vi "BonOMM-SAOMM.Test.vi"() -> ()   [LabVIEW 2011] (continued)
                        n4610 = Subtract(x=w3202, y=w3207) -> (x-y=w3206:dbl)
                        n4611 = Absolute Value(x=w3206) -> (abs(x)=w3205:dbl)
                        n4612 = Greater?(x=w3205, y=2.0) -> (0:w3203:bool)
                        n4613 = And(x=w3208, y=w3203) -> (x .and. y?=w3209:bool)
                        n4614 = case shown="True" w3209 {
                          tunnel: w3202 -> [_ w3214]
                          frame False {
                          }
                          frame True {
                            n4615 = local read "Foyer à 0°"() -> (w3213:i32)
                            n4616 = local read "Ath_coef"() -> (w3211:dbl)
                            n4617 = To Double Precision Float(number=w3213) -> (double precision float=w3212:dbl)
                            n4618 = call "Athermalize-focus.vi"("Coefficient Thermique"=w3211, "temperature actuelle"=w3214, "Foyer à 0°"=w3212) -> ("Foyer suggérer"=w3210:i32)  [unwired: 1 in]
                            n4619 = Number To Decimal String(number=w3210) -> (decimal integer string=w3223:string)  [unwired: 1 in]
                            n4620 = Concatenate Strings("La température a suffisamment changée\npour justifier un ajustement du foyer ...\nDésirez-vous faire l'ajustement maintenant ?\n(Valeur suggérée : " ("message"), w3223, " ADU)" ("string")) -> (w3221:string)
                            n4621 = call <vilib>:"Three Button Dialog.vi"("Allow user to close window? (TRUE)"=FALSE, "Justify Message (Left)"=enum16{"Left", "Center", "Right"}."Center", "Right Button Text (\"Cancel\")"="Ne plus me demander" ("string"), "Center Button Text (\"No\")"="NON" ("string"), "Left Button Text (\"Yes\")"="OUI" ("string"), "message"=w3221) -> ("Which Button?"=w3220:T59)  [unwired: 5 in]
                            n4622 = case shown="\"Center Button\"" w3220 {
                              frame "Left Button", Default {
                              }
                              frame "Center Button" {
                                n4623 = local read "indic-T-struct"() -> (w3225:dbl)
                                n4624 = local write "tmp.str"(w3225) -> ()
                              }
                              frame "Right Button" {
                                "Bypass Auto-focus" <- TRUE ("Allow user to close window? (TRUE)")
                              }
                            }
                          }
                        }
                      }
                    }
                  }
                }
                n4625 = Quotient & Remainder(x=w3171, y=10) -> (x-y*floor(x/y)=w3173:i32)  [unwired: 1 out]
                n4626 = Equal To 0?(x=w3173) -> (x = 0?=w3170:bool)
                n4627 = case shown="False" w3170 {
                  frame False {
                  }
                  frame True {
                    n4628 = disable-structure shown="Enabled" {
                      frame Disabled {
                        n4629 = call "DCON-Read.vi"("VRN in"="HexTemp VRN") -> ("DataCluster"=→"Hexapode Temperatures":T13, "Boolean array"=→"Hexapod Alarms":bool[], "error out"=w3177:errorcluster)  [unwired: 11 in, 1 out]
                        n4630 = local write "HexapodeTempError"(w3177) -> ()
                        n4631 = Unbundle By Name(w3177) -> ("status"=w3180:bool)
                        n4632 = Not(x=w3180) -> (.not. x?=→"HexTemp COMM":bool)
                      }
                      frame Enabled {
                      }
                    }
                  }
                }
              }
              event "Setting", "Focus slew": Value Change {
                n4633 = event-data() -> ()  [unwired: 1 in, 6 out]
                n4634 = local read "Focus slew"() -> (w3229:bool)
                n4635 = local read "Setting"() -> (w3231:bool)
                n4636 = Not(x=w3229) -> (.not. x?=w3228:bool)
                n4637 = case shown="False" w3231 {
                  selector: w3231 -> [_ w3237]
                  tunnel: [w3232 w3237] -> w3230
                  frame False {
                    n4638 = local read "Foyer"() -> (w3235:dbl)
                    n4639 = local read "Foyer Nominal"() -> (w3236:dbl)
                    n4640 = Subtract(x=w3236, y=w3235) -> (x-y=w3234:dbl)
                    n4641 = Greater?(x=w3234, y=1.0) -> (0:w3232:bool)
                  }
                  frame True {
                  }
                }
                n4642 = And(x=w3228, y=w3230) -> (x .and. y?=w3227:bool)
                n4643 = case shown="False" w3227 {
                  frame False {
                    # "Ici, normalement, on est à la fin d'une séquence de foyer ..."
                    n4644 = local read "Foyer"() -> (w3238:dbl)
                    n4645 = Get Date/Time In Seconds() -> (seconds since 1Jan1904=w3240:timestamp)
                    n4646 = To Extended Precision Float(1:w3240) -> (0:→"last_foc_chg":ext)
                    n4647 = local write "Foyer Nominal"(w3238) -> ()
                    n4648 = local read "indic-T-struct"() -> (→"tmp.str":dbl)
                    "CheckFocus" <- TRUE
                  }
                  frame True {
                  }
                }
              }
              event "Recalculer": Value Change {
                # "Ne devrait pas être fait sur une base régulière, mais simplement quand les paramètres ont changés ...\n\nC'est ici qu'on veut cleaner les dossiers de data et construire les mosaiques d'image et de données !!!\n\nPour l'instant, tout a été arraché le temps de débuggé les Queries USNO & DSS !!!"
                n4649 = event-data() -> ()  [unwired: 1 in, 6 out]
                n4650 = case shown="True" "Recalculer" {
                  selector: "Recalculer" -> [_ w3250]
                  frame False {
                  }
                  frame True {
                    n4651 = stacked-sequence {
                      seq-local: [w3257 _ _ _] -> [_ w3261 w3289 _]
                      seq-local: [w3256 _ _ _] -> [_ w3262 w3288 _]
                      tunnel: w3250 -> [_ _ _ _]
                      frame #0 {
                        w3258 = FALSE ("DSS_ready")
                        # "Époque DSS et USNO"
                        # "Ici il faudra s'assurer que l'astrométrie tourne autour du centre, mais\nutilise la position synchronisée comme valeur de référence"
                        # "Ces variables sont probablement\nmaintenant inutiles"
                        # "à remettre éventuellement ..."
                        # "Calcul les paramètres du champ ..."
                        n4652 = disable-structure shown="Disabled" {
                          frame Disabled {
                          }
                          frame Enabled {
                          }
                        }
                        n4653 = local read "Img DEC"() -> (w3253:dbl)
                        n4654 = local read "Img RA"() -> (w3252:dbl)
                        n4655 = local read "Epoch Tel"() -> (w3255:dbl)
                        n4656 = call "precess.vi"("Eq2"=2000.0, "Eq1"=w3255, "DEC 1"=w3253, "RA 1"=w3252) -> ("DEC 2"=w3257:dbl, "RA 2"=w3256:dbl)
                        n4657 = local write "USNO_ready"(FALSE) -> ()
                        n4658 = local write "Indicateur d'état"("Calcul des paramètres du champ") -> ()
                        "DSS_ready" <- w3258
                        "USNO_ready" <- w3258
                      }
                      frame #1 {
                        # "Télécharge les données USNO associées ..."
                        # "DEC centre img"
                        # "RA centre img"
                        n4659 = flat-sequence {
                          tunnel: w3262 -> [w3272]
                          tunnel: w3261 -> [w3271]
                          tunnel: [w3266] -> w3260
                          tunnel: w3260 -> [w3284]
                          frame #0 {
                            # "R1mag limite USNO"
                            n4660 = local read "Représentation"() -> (w3263:dbl)
                            n4661 = local read "path_data"() -> (w3268:path)
                            n4662 = while {
                              stop <- w3274 stop-if-true
                              n4663 = local read "BestTargetLed"() -> (w3276:bool)
                              n4664 = Wait (ms)(milliseconds to wait=u32 333) -> ()  [unwired: 1 out]
                              n4665 = Not(x=w3276) -> (.not. x?=w3275:bool)
                              n4666 = local write "BestTargetLed"(w3275) -> ()
                              n4667 = local read "USNO_ready"() -> (w3274:bool)
                            }
                            n4668 = local read "wgetexec"() -> (w3267:path)
                            n4669 = call "QueryUSNO.vi"("wget"=w3267, "Data dir Path"=w3268, "mag_limit"=12.0, "radius"=w3263, "DEC"=w3271, "RA"=w3272) -> ("Data OUT"=w3269:string[][], "No Error"=w3264:bool)  [unwired: 3 in, 1 out]
                            n4670 = case shown="True" w3264 {
                              tunnel: w3269 -> [_ w3283]
                              tunnel: w3264 -> [w3278 w3280]
                              tunnel: [w3278 w3280] -> w3266
                              tunnel: [TRUE TRUE] -> w3265
                              frame False {
                              }
                              frame True {
                                # "6 = R1mag"
                                n4671 = call "Sort_USNO_data.vi"("Column Used"=6, "Data IN"=w3283) -> ("Data OUT"=→"USNO_data":string[][])  [unwired: 8 in, 1 out]
                              }
                            }
                            n4672 = local write "USNO_ready"(w3265) -> ()
                          }
                          frame #1 {
                            n4673 = local write "USNO_ready"(w3284) -> ()
                            n4674 = local write "BestTargetLed"(w3284) -> ()
                          }
                        }
                      }
                      frame #2 {
                        # "Pour que l'image disparaisse quand\non coche ou décoche l'option du menu"
                        # "Get the dss image ...\nÉventuellement va vérifier l'existence et créer les mosaïques\nPour l'instant, on ne le permet qu'avec le bouton \"GetDSS\""
                        n4675 = local read "Img RA"() -> (w3299:dbl)
                        n4676 = local read "imageDSS"() -> (w3286:bool)
                        n4677 = local read "Img DEC"() -> (w3290:dbl)
                        n4678 = Subtract(x=w3288, y=w3299) -> (x-y=w3297:dbl)
                        n4679 = Subtract(x=w3289, y=w3290) -> (x-y=w3298:dbl)
                        n4680 = Absolute Value(x=w3297) -> (abs(x)=w3296:dbl)
                        n4681 = Absolute Value(x=w3298) -> (abs(x)=w3295:dbl)
                        n4682 = Greater?(x=w3296, y=1.0) -> (0:w3291:bool)
                        n4683 = Not(x=w3286) -> (.not. x?=w3285:bool)
                        n4684 = Greater?(x=w3295, y=1.0) -> (0:w3292:bool)
                        n4685 = Compound Arithmetic op=OR(w3291, w3292, w3285) -> (w3287:bool)
                        n4686 = case shown="True" w3287 {
                          tunnel: w3288 -> [_ w3302]
                          tunnel: w3289 -> [_ w3303]
                          frame False {
                            n4687 = local read "imageDSS"() -> (w3300:bool)
                            n4688 = local write "DSS_ready"(w3300) -> ()
                          }
                          frame True {
                            n4689 = local read "imageDSS"() -> (w3301:bool)
                            n4690 = case shown="True" w3301 {
                              tunnel: w3303 -> [_ w3308]
                              tunnel: w3302 -> [_ w3307]
                              frame False {
                                n4691 = property on="TableXYPos" class="XYGraph (strict)"("PlotImages.Back"=picture data[5B] ("Images")) -> ()  [unwired: 2 in, 2 out]
                              }
                              frame True {
                                n4692 = flat-sequence {
                                tunnel: w3307 -> [w3318]
                                tunnel: w3308 -> [w3319]
                                tunnel: [w3319] -> w3306
                                tunnel: [w3318] -> w3305
                                tunnel: w3306 -> [w3328]
                                tunnel: w3305 -> [w3327]
                                frame #0 {
                                w3309 = u16 1 items=["Region d'intérêt", "Prévisualisation"] ("ImageUsage")
                                w3314 = 0
                                n4693 = Initialize Array(sgl 0.0, w3314, w3314) -> (w3313:sgl[][])
                                n4694 = local write "ImgData"(w3313) -> ()
                                n4695 = local write "SubIMG4DSS?"(TRUE ("SubIMG4DSS?")) -> ()
                                n4696 = local write "ImgAstrom"(T4 {"NAXIS"=[], "CD"=[], "CDELT"=[], "CRPIX"=[], "CTYPE"=[], "CRVAL"=[], "LONGPOLE"=180.0, "LATPOLE"=90.0, "PV2"=[]} ("ImgAstrom")) -> ()
                                n4697 = call "Draw_crosshair.vi"("Image IN"=w3313, "White Value"=sgl 255.0) -> ("Image OUT"=w3312:sgl[][])  [unwired: 13 in]
                                n4698 = property on="TableXYPos" class="XYGraph (strict)"("PlotImages.Back"=picture data[5B] ("Images")) -> ()  [unwired: 2 in, 2 out]
                                n4699 = local write "subimg"(w3312) -> ()
                                n4700 = local write "ImageUsage"(w3309) -> ()
                                }
                                frame #1 {
                                # "Ici, le code devrait vérifier l'existence des images sur le disque ..."
                                n4701 = local read "Représentation"() -> (w3322:dbl)
                                n4702 = local read "path_dss"() -> (w3325:path)
                                n4703 = local read "wgetexec"() -> (w3324:path)
                                n4704 = Add(x=4.0, y=w3322) -> (x+y=w3320:dbl)
                                n4705 = call "Query_Vizier.vi"("Folder"=w3325, "wget"=w3324, "Width"=w3320, "Height"=w3320, "DEC"=w3328, "RA"=w3327) -> ("error?"=w3323:bool, "Path2Image"=w3331:path)  [unwired: 4 in]
                                "Path2Image" <- w3331
                                n4706 = case shown="False" w3323 {
                                tunnel: w3327 -> [w3336 _]
                                tunnel: w3328 -> [w3335 _]
                                tunnel: w3331 -> [w3338 _]
                                tunnel: [w3336 -inf ("RA OUT")] -> w3330
                                tunnel: [w3335 -inf ("RA OUT")] -> w3329
                                tunnel: [TRUE FALSE] -> w3326
                                frame False {
                                # "ImgData et ImgAstrom\nsont lié à plus grand que le\nchamp affiché."
                                n4707 = local read "FieldAstrom"() -> (w3334:T4)
                                n4708 = property on="TableXYPos" class="XYGraph (strict)"() -> ("Height"=w3344:u32, "Width"=w3343:u32)  [unwired: 2 in, 2 out]
                                n4709 = property on="TableXYPos" class="XYGraph (strict)"() -> ("XScale.Range"=w3340:T26, "YScale.Range"=w3339:T26)  [unwired: 2 in, 2 out]
                                n4710 = To Long Integer(number=w3344) -> (32bit integer=w3342:i32)
                                n4711 = To Long Integer(number=w3343) -> (32bit integer=w3341:i32)
                                n4712 = call "Draw_graph_background.vi"("Y Scale.Range"=w3339, "ImgRA"=w3336, "X Scale.Range"=w3340, "ImgDEC"=w3335, "Field Astrometry"=w3334, "New Width"=w3341, "New Height"=w3342, "path"=w3338) -> ("ImgData"=→"ImgData":sgl[][], "Astrometry"=→"ImgAstrom":T4, "Images"=w3333:picture)  [unwired: 1 out]
                                n4713 = property on="TableXYPos" class="XYGraph (strict)"("PlotImages.Back"=w3333) -> ()  [unwired: 2 in, 2 out]
                                }
                                frame True {
                                }
                                }
                                "Img RA" <- w3330
                                "Img DEC" <- w3329
                                n4714 = local write "DSS_ready"(w3326) -> ()
                                }
                                }
                              }
                            }
                          }
                        }
                      }
                      frame #3 {
                        # "Retrace l'image de la caméra de référence ..."
                        n4715 = local write "Recalculer"(FALSE ("Recalculer")) -> ()
                      }
                    }
                  }
                }
                n4716 = while {
                  tunnel: [FALSE] -> w3243
                  stop <- w3249 continue-if-true
                  n4717 = local read "Downloading ..."() -> (w3247:bool)
                  n4718 = Not(x=w3247) -> (.not. x?=→"Downloading ...":bool)
                  n4719 = Wait (ms)(milliseconds to wait=u32 333) -> ()  [unwired: 1 out]
                  n4720 = local read "Recalculer"() -> (w3249:bool)
                }
                n4721 = local write "Downloading ..."(w3243) -> ()
              }
              event "Slewing": Value Change {
                n4722 = event-data() -> ("NewVal"=w3350:bool)  [unwired: 1 in, 5 out]
                n4723 = case shown="False" w3350 {
                  frame False {
                    w3352 = FALSE ("Blinking")
                    w3353 = 0
                    # "Fin d'un déplacement ..."
                    # "Activer les boutons"
                    n4724 = property on="GO" class="Bool (strict)"("Disabled"=w3353) -> ()  [unwired: 2 in, 2 out]
                    n4725 = property on="Synctel" class="Bool (strict)"("Disabled"=w3353) -> ()  [unwired: 2 in, 2 out]
                    n4726 = property on="ModifRotation" class="Bool (strict)"("Disabled"=w3353) -> ()  [unwired: 2 in, 2 out]
                    n4727 = property on="Offset OK" class="Bool (strict)"("Disabled"=w3353) -> ()  [unwired: 2 in, 2 out]
                    n4728 = property on="ModifFoyer" class="Bool (strict)"("Disabled"=w3353) -> ()  [unwired: 2 in, 2 out]
                    n4729 = property on="Écran" class="Bool (strict)"("Disabled"=w3353) -> ()  [unwired: 2 in, 2 out]
                    n4730 = property on="Zénith" class="Bool (strict)"("Disabled"=w3353) -> ()  [unwired: 2 in, 2 out]
                    n4731 = property on="Range" class="Bool (strict)"("Disabled"=w3353) -> ()  [unwired: 2 in, 2 out]
                    n4732 = property on="Zénith" class="Bool (strict)"("Blinking"=w3352) -> ()  [unwired: 2 in, 2 out]
                    n4733 = property on="Range" class="Bool (strict)"("Blinking"=w3352) -> ()  [unwired: 2 in, 2 out]
                    n4734 = property on="Écran" class="Bool (strict)"("Blinking"=w3352) -> ()  [unwired: 2 in, 2 out]
                    n4735 = property on="ModCoor" class="Bool (strict)"("Disabled"=w3353) -> ()  [unwired: 2 in, 2 out]
                    n4736 = property on="ModifDome" class="Bool (strict)"("Disabled"=w3353) -> ()  [unwired: 2 in, 2 out]
                    n4737 = local read "Déplacement usager"() -> (w3351:bool)
                    n4738 = case shown="True" w3351 {
                      frame False {
                        w3354 = FALSE ("Déplacement usager")
                        n4739 = local write "Déplacement usager"(w3354) -> ()
                        n4740 = local write "From library"(w3354) -> ()
                      }
                      frame True {
                        w3363 = "\t"
                        w3369 = "_"
                        w3375 = TRUE ("replace all? (F)")
                        w3376 = " "
                        w3377 = "0"
                        w3380 = i16 2 ("width (-)")
                        w3381 = i16 0 ("width (-)")
                        # "Devrait aussi être mis dans un log pour pouvoir y revenir plus tard ..."
                        # "Enregistre la nouvelle position du télescope"
                        n4741 = local write "Déplacement usager"(FALSE ("Déplacement usager")) -> ()
                        n4742 = local read "Epoch Tel"() -> (w3385:dbl)
                        n4743 = local read "DEC Tel"() -> (w3383:dbl)
                        n4744 = local read "RA Tel"() -> (w3384:dbl)
                        n4745 = call "time-sec-to-time-str-DEC.vi"("Numeric"=w3384) -> ("formatted-str"=w3366:string)
                        n4746 = call "time-sec-to-time-str-DEC.vi"("Numeric"=w3383) -> ("formatted-str"=w3365:string)
                        n4747 = Number To Fractional String(number=w3385, width (-)=i16 4, precision (6)=i16 2) -> (F-format string=w3364:string)  [unwired: 1 in]
                        n4748 = Get Date/Time String() -> (time string=w3367:string)  [unwired: 3 in, 1 out]
                        n4749 = local read "From library"() -> (w3389:bool)
                        n4750 = Concatenate Strings(w3367, w3363, w3366, w3363, w3365, w3363, w3364, "\r\n") -> (w3355:string)
                        n4751 = call "GetUTC.vi"() -> ("Day"=w3359:dbl, "Month"=w3360:dbl, "Year"=w3361:dbl)  [unwired: 6 out]
                        n4752 = case shown="True" w3389 {
                          tunnel: [FALSE FALSE] -> w3388
                          tunnel: w3366 -> [w3394 w3401]
                          tunnel: w3365 -> [w3393 w3402]
                          tunnel: w3364 -> [w3392 w3403]
                          tunnel: w3367 -> [w3391 w3400]
                          frame False {
                            w3396 = i16 0 items=["tel coords", "tel offset", "guidage"] ("options")
                            n4753 = local read "Obslib"() -> (w3397:string[][])
                            n4754 = Build Array(w3394, w3393, w3392, w3391) -> (w3398:string[])
                            n4755 = call "Coords to chart(new).vi"("DataLine"=w3398, "options"=w3396, "Tableau entrant"=w3397) -> ("historique"=w3399:string[][])
                            n4756 = local write "Obslib"(w3399) -> ()
                          }
                          frame True {
                            w3405 = i16 0 items=["tel coords", "tel offset", "guidage"] ("options")
                            n4757 = local read "Obslib"() -> (w3406:string[][])
                            n4758 = Build Array(w3401, w3402, w3403, w3400) -> (w3407:string[])
                            n4759 = call "Coords to chart(new).vi"("DataLine"=w3407, "options"=w3405, "Tableau entrant"=w3406) -> ("historique"=w3408:string[][])
                            n4760 = local write "Obslib"(w3408) -> ()
                          }
                        }
                        "From library" <- w3388
                        n4761 = Number To Fractional String(number=w3361, width (-)=i16 4, precision (6)=w3381) -> (F-format string=w3374:string)  [unwired: 1 in]
                        n4762 = Number To Fractional String(number=w3360, width (-)=w3380, precision (6)=w3381) -> (F-format string=w3379:string)  [unwired: 1 in]
                        n4763 = Number To Fractional String(number=w3359, width (-)=w3380, precision (6)=w3381) -> (F-format string=w3378:string)  [unwired: 1 in]
                        n4764 = Search and Replace String(replace all?=w3375, input string=w3379, search string=w3376, replace string=w3377) -> (result string=w3373:string)  [unwired: 4 in, 3 out]
                        n4765 = Search and Replace String(replace all?=w3375, input string=w3378, search string=w3376, replace string=w3377) -> (result string=w3372:string)  [unwired: 4 in, 3 out]
                        n4766 = local read "path_pointing"() -> (w3371:path)
                        n4767 = Concatenate Strings(w3374, w3369, w3373, w3369, w3372, ".pnt") -> (w3370:string)
                        n4768 = Build Path(base path=w3371, name or relative path=w3370) -> (appended path=w3356:path)
                        n4769 = local read "File I/O Error"() -> (w3358:errorcluster)
                        n4770 = call "PNT-Data-Write.vi"("Path IN"=w3356, "Data Line"=w3355, "Error IN"=w3358) -> ("Error OUT"=w3357:errorcluster)  [unwired: 11 in, 1 out]
                        n4771 = local write "File I/O Error"(w3357) -> ()
                      }
                    }
                  }
                  frame True {
                    w3409 = 2
                    # "Début d'un déplacement"
                    # "Désactiver les boutons de TCS"
                    n4772 = property on="GO" class="Bool (strict)"("Disabled"=w3409) -> ()  [unwired: 2 in, 2 out]
                    n4773 = property on="ModifFoyer" class="Bool (strict)"("Disabled"=w3409) -> ()  [unwired: 2 in, 2 out]
                    n4774 = property on="Écran" class="Bool (strict)"("Disabled"=w3409) -> ()  [unwired: 2 in, 2 out]
                    n4775 = property on="ModCoor" class="Bool (strict)"("Disabled"=w3409) -> ()  [unwired: 2 in, 2 out]
                    n4776 = property on="Zénith" class="Bool (strict)"("Disabled"=w3409) -> ()  [unwired: 2 in, 2 out]
                    n4777 = property on="Range" class="Bool (strict)"("Disabled"=w3409) -> ()  [unwired: 2 in, 2 out]
                    n4778 = property on="Synctel" class="Bool (strict)"("Disabled"=w3409) -> ()  [unwired: 2 in, 2 out]
                    n4779 = property on="ModifRotation" class="Bool (strict)"("Disabled"=w3409) -> ()  [unwired: 2 in, 2 out]
                    n4780 = property on="Offset OK" class="Bool (strict)"("Disabled"=w3409) -> ()  [unwired: 2 in, 2 out]
                    n4781 = property on="ModifDome" class="Bool (strict)"("Disabled"=w3409) -> ()  [unwired: 2 in, 2 out]
                  }
                }
              }
            }
            n4782 = local read "Quit"() -> (w3167:bool)
          }
          "Événements Software" <- w952
          n4783 = while {
            tunnel: [w1226] -> w950
            stop <- w1226 stop-if-true
            # "Boucle périodique pour PrAMS + Hexapode + LVDTs\nÉvénements lents ..."
            n4784 = stacked-sequence {
              frame #0 {
                n4785 = disable-structure shown="Disabled" {
                  frame Disabled {
                    n4786 = local read "LVDT-RA"() -> (w1230:refnum<k21>)
                    n4787 = local read "LVDT Error"() -> (w1229:errorcluster)
                    n4788 = Unbundle By Name(w1229) -> ("status"=w1228:bool)
                    n4789 = case shown="False" w1228 {
                      tunnel: w1230 -> [w1243 _]
                      tunnel: w1229 -> [_ _]
                      frame False {
                        n4790 = call "Read-LVDT-Data.vi"("shared variable refnum"=w1243, "MaxLen"=631 ("timeout ms"), "Data IN"="LVDT-RA-Data") -> ("Graph Data"=w1237:dbl[], "Data OUT"=w1239:dbl[], "error out"=→"LVDT Error":errorcluster)  [unwired: 10 in]
                        "Graph Data" <- w1237
                        n4791 = local write "LVDT-RA-Data"(w1239) -> ()
                        n4792 = Subtract(x=w1237, y="LVDT-zero") -> (x-y=w1244:dbl[])
                        n4793 = Multiply(x="LVDT-scale", y=w1244) -> (x*y=w1234:dbl[])
                        n4794 = Array Size(array=w1234) -> (size(s)=w1233:i32)
                        n4795 = Decrement(x=w1233) -> (x-1=w1231:i32)
                        n4796 = Bundle(0.0, "LVDT-time"="LVDT-time", w1234) -> (→"LVDT-RA-coarse" →"LVDT-RA-closeup":cluster{dbl, "LVDT-time":dbl, dbl[]})  [unwired: 1 in]
                        n4797 = Index Array(array=w1234, index=w1231) -> (element=→"LVDT-RA-inst":dbl)
                      }
                      frame True {
                      }
                    }
                  }
                  frame Enabled {
                  }
                }
              }
              frame #1 {
                # "Si la communication avec TCS et PrAMS sont actives, on update les valeurs de ALT/AZ/ROT de Prams\n\nN.B. : L'erreur associée (#64) : est ignorée par la boucle \"emterror\" ci-bas ..."
                n4798 = local read "PrAMS COMM"() -> (w1248:bool)
                n4799 = local read "TCS COMM"() -> (w1249:bool)
                n4800 = And(x=w1249, y=w1248) -> (x .and. y?=w1247:bool)
                n4801 = case shown="False" w1247 {
                  frame False {
                  }
                  frame True {
                    n4802 = local read "Epoch Tel"() -> (w1263:dbl)
                    n4803 = local read "RA Tel"() -> (w1267:dbl)
                    n4804 = local read "DEC Tel"() -> (w1266:dbl)
                    n4805 = local read "AnnéeRL"() -> (w1262:dbl)
                    n4806 = local read "LST"() -> (w1261:dbl)
                    n4807 = call "ad2deg.vi"("DEC (sec)"=w1266, "RA (sec)"=w1267) -> ("DEC (°)"=w1264:dbl, "RA (°)"=w1265:dbl)
                    n4808 = call "ad2deg.vi"("RA (sec)"=w1261) -> ("RA (°)"=w1260:dbl)  [unwired: 1 in, 1 out]
                    n4809 = call "precess.vi"("Eq2"=w1262, "Eq1"=w1263, "DEC 1"=w1264, "RA 1"=w1265) -> ("DEC 2"=w1258:dbl, "RA 2"=w1268:dbl)
                    "DEC" <- w1258
                    n4810 = Subtract(x=w1260, y=w1268) -> (x-y=w1259:dbl)
                    "HA" <- w1259
                    n4811 = control-ref of="PrAMS-ACK"() -> (w1253:refnum<vi>)
                    n4812 = control-ref of="PrAMS actif"() -> (w1252:refnum<vi>)
                    n4813 = local read "PrAMS VRN"() -> (w1254:refnum<visa-resource-name>)
                    n4814 = local read "PrAMS Error"() -> (w1255:errorcluster)
                    n4815 = local read "Signature"() -> (w1257:u32)
                    n4816 = local read "MessageType"() -> (w1256:cluster{string[], u32[]})
                    n4817 = call "SAOMM-SetTelescopeProperties.vi"("PRAMMS-COMM IN"=w1254, "PramsActif"=w1252, "PrAMS-ACK"=w1253, "HA"=w1259, "DEC"=w1258, "Error IN"=w1255, "Signature"=w1257, "MsgTypeEnum"=w1256) -> ("PRAMMS-COMM OUT"=w1250:refnum<visa-resource-name>, "Error OUT"=w1251:errorcluster)  [unwired: 6 in]
                    n4818 = local write "PrAMS VRN"(w1250) -> ()
                    n4819 = local write "PrAMS Error"(w1251) -> ()
                  }
                }
              }
              frame #2 {
                # "L'angle ne peut être envoyé que si l'asservissement est OFF"
                n4820 = local read "Servo"() -> (w1269:bool)
                n4821 = case shown="False" w1269 {
                  frame False {
                    # "Prams à un 180° dans sa matrice d'Euler"
                    n4822 = local read "RotationEffective"() -> (w1280:dbl)
                    n4823 = local read "PrAMS VRN"() -> (w1275:refnum<visa-resource-name>)
                    n4824 = control-ref of="PrAMS-ACK"() -> (w1272:refnum<vi>)
                    n4825 = local read "PrAMS Error"() -> (w1276:errorcluster)
                    n4826 = local read "MessageType"() -> (w1277:cluster{string[], u32[]})
                    n4827 = control-ref of="PrAMS actif"() -> (w1273:refnum<vi>)
                    n4828 = local read "Signature"() -> (w1274:u32)
                    n4829 = call "Fix_angle.vi"("±180 -> 0-360?"=FALSE, "Angle IN"=w1280) -> ("Angle OUT"=w1279:dbl)  [unwired: 3 in]
                    n4830 = Negate(x=w1279) -> (-x=w1270:dbl)
                    n4831 = call-poly "SAOMM-Num2littleEndian.vi"("Number"=w1270) -> ("LiitleEndianedData"=w1278:u8[])  [unwired: 14 in]
                    n4832 = call "SAOMM-SendSET.vi"("PRAMMS-COMM IN"=w1275, "Active Refnum"=w1273, "PrAMS-ACK"=w1272, "Signature"=w1274, "Error IN"=w1276, "MessageType"=w1277, "Active SET"="emtSetMountingPlateAngle", "Value (little endianed byte array)"=w1278) -> ()  [unwired: 4 in, 4 out]
                  }
                  frame True {
                  }
                }
              }
              frame #3 {
                # "Enregistre environ 2 fois par \"Considered Lenght\""
                # "Update l'historique de guidage et enregistre log dans un fichier ..."
                n4833 = local read "Graph-Centroids"() -> (w1284:cluster{"TimeArray":dbl[], dbl[]}[])
                n4834 = Index Array(array=w1284) -> (element #1=w1301:cluster{"TimeArray":dbl[], dbl[]}, element #2=w1300:cluster{"TimeArray":dbl[], dbl[]})  [unwired: 2 in]
                n4835 = Unbundle(w1301) -> (w1298:dbl[])  [unwired: 1 out]
                n4836 = Unbundle(w1300) -> ("TimeArray"=w1283:dbl[], w1299:dbl[])
                n4837 = local read "LastSaveTimeStamp"() -> (w1290:dbl)
                n4838 = local read "ConsideredLenght"() -> (w1294:i32)
                n4839 = call "TimeStamp-Extractor.vi"("TimeStampArray"=w1283) -> ("LastTimestamp"=w1289:dbl)  [unwired: 12 in, 2 out]
                n4840 = To Double Precision Float(number=w1294) -> (double precision float=w1293:dbl)
                n4841 = call "Guide_error_histo.vi"("X Array"=w1298, "intervals"=11, "Y array"=w1299, "limite haute"=5.0, "limite basse"=-5.0 ("limite haute")) -> ("XY graph"=→"Guiderreur":cluster{dbl[], dbl[]}[])  [unwired: 1 out]
                n4842 = local read "CentroidsData"() -> (w1285:cluster{dbl[], dbl[]}[])
                n4843 = expression code="x/2"(w1293) -> (w1292:dbl)
                n4844 = Add(x=w1290, y=w1292) -> (x+y=w1291:dbl)
                n4845 = Greater?(x=w1289, y=w1291) -> (0:w1287:bool)
                n4846 = Or(x="ForceSaveToFile", y=w1287) -> (x .or. y?=w1288:bool)
                n4847 = case shown="True" w1288 {
                  tunnel: w1289 -> [_ w1328]
                  tunnel: w1290 -> [_ w1313]
                  tunnel: w1285 -> [_ w1329]
                  frame False {
                  }
                  frame True {
                    # "Va peut-être perdre les quelques minutes juste avant la fermeture \n... pour ce que ça changera c'est beaucoup de travail."
                    n4848 = local read "path_trackfile"() -> (w1312:path)
                    n4849 = Strip Path(path=w1312) -> (stripped path=w1306:path)  [unwired: 1 out]
                    n4850 = local read "path_trackfile"() -> (w1326:path)
                    n4851 = Build Path(base path=w1306, name or relative path="Hexapod") -> (appended path=w1304:path)
                    n4852 = call "GetPathFromTimeStamp.vi"("UTC Time"=FALSE, "LocalTimeStamp"=w1313, "Changement de date à midi ?"=TRUE) -> ("Date String"=w1302:string)  [unwired: 11 in, 1 out]
                    n4853 = call "CheckAndCreateDirectory.vi"("Path IN"=w1304) -> ("Path OUT"=w1303:path, "Exists?"=w1309:bool, "Created?"=w1308:bool)  [unwired: 12 in]
                    n4854 = call "GetPathFromTimeStamp.vi"("UTC Time"=TRUE, "LocalTimeStamp"=w1328, "Changement de date à midi ?"=TRUE) -> ("Date String"=w1327:string)  [unwired: 11 in, 1 out]
                    n4855 = local read "ForceSaveToFile"() -> (w1318:bool)
                    n4856 = Build Path(base path=w1326, name or relative path=w1327) -> (appended path=w1325:path)
                    n4857 = Or(x=w1309, y=w1308) -> (x .or. y?=w1307:bool)
                    n4858 = local read "Servo"() -> (w1317:bool)
                    n4859 = case shown="True" w1307 {
                      tunnel: w1313 -> [_ w1336]
                      tunnel: w1303 -> [_ w1335]
                      tunnel: w1302 -> [_ w1333]
                      frame False {
                      }
                      frame True {
                        # "Log de l'hexapode"
                        n4860 = Concatenate Strings(w1333, ".hex") -> (w1331:string)
                        n4861 = local read "HexXData"() -> (w1338:cluster{dbl[], dbl[]}[])
                        n4862 = local read "HexYData"() -> (w1337:cluster{dbl[], dbl[]}[])
                        n4863 = local read "CumulativeError"() -> (w1330:cluster{dbl[], dbl[]}[])
                        n4864 = Build Path(base path=w1335, name or relative path=w1331) -> (appended path=w1334:path)
                        n4865 = call "LogHexapodData.vi"("LogFilePath"=w1334, "TimeStampTreshold"=w1336, "X IN"=w1338, "Y IN"=w1337, "Cumul IN"=w1330) -> ()  [unwired: 10 in, 1 out]
                      }
                    }
                    n4866 = call "CheckAndCreateDirectory.vi"("Path IN"=w1325) -> ("Path OUT"=w1322:path, "Exists?"=w1324:bool, "Created?"=w1323:bool)  [unwired: 12 in]
                    n4867 = Or(x=w1324, y=w1323) -> (x .or. y?=w1320:bool)
                    n4868 = Or(x=w1317, y=w1318) -> (x .or. y?=w1316:bool)
                    n4869 = local read "TrackLogFilename"() -> (w1321:string)
                    n4870 = And(x=w1320, y=w1316) -> (x .and. y?=w1319:bool)
                    n4871 = case shown="True" w1319 {
                      tunnel: w1329 -> [_ w1348]
                      tunnel: w1313 -> [_ w1345]
                      tunnel: w1322 -> [_ w1344]
                      tunnel: w1321 -> [_ w1342]
                      frame False {
                      }
                      frame True {
                        # "Log de guidage"
                        n4872 = local read "SNRData"() -> (w1340:cluster{dbl[], dbl[]}[])
                        n4873 = local read "FluxData"() -> (w1339:cluster{dbl[], dbl[]}[])
                        n4874 = Build Path(base path=w1344, name or relative path=w1342) -> (appended path=w1343:path)
                        n4875 = local write "ForceSaveToFile"(FALSE ("ForceSaveToFile")) -> ()
                        n4876 = local read "Dec Sonde"() -> (w1347:dbl)
                        n4877 = local read "RA Sonde"() -> (w1346:dbl)
                        n4878 = call "LogSourceData.vi"("LogFilePath"=w1343, "DECsonde"=w1347, "RAsonde"=w1346, "TimeStampTreshold"=w1345, "SNR IN"=w1340, "Flux IN"=w1339, "Centroids IN"=w1348) -> ()  [unwired: 8 in, 1 out]
                      }
                    }
                    "LastSaveTimeStamp" <- w1328
                  }
                }
              }
              frame #4 {
                n4879 = local read "LastProcID"() -> (w1360:u64)
                n4880 = local read "LastProcSavedID"() -> (w1361:u64)
                n4881 = Get Date/Time In Seconds() -> (seconds since 1Jan1904=w1352:timestamp)
                n4882 = local read "FalconProcTimeStamp"() -> (w1355:dbl)
                n4883 = local read "ConsideredLenght"() -> (w1356:i32)
                n4884 = To Double Precision Float(number=w1352) -> (double precision float=w1351:dbl)
                n4885 = Greater?(x=w1360, y=w1361) -> (0:w1359:bool)
                n4886 = To Double Precision Float(number=w1356) -> (double precision float=w1357:dbl)
                n4887 = Add(x=w1355, y=w1357) -> (x+y=w1354:dbl)
                n4888 = Greater?(x=w1351, y=w1354) -> (0:w1353:bool)
                n4889 = And(x=w1359, y=w1353) -> (x .and. y?=w1349:bool)
                n4890 = Or(x="SaveFalconProc", y=w1349) -> (x .or. y?=w1358:bool)
                n4891 = case shown="True" w1358 {
                  tunnel: w1360 -> [_ w1363]
                  tunnel: w1351 -> [_ w1362]
                  frame False {
                  }
                  frame True {
                    # "Demande d'enregistre de la prochaine trame FalconProcessed"
                    n4892 = local read "path_data"() -> (w1367:path)
                    n4893 = local read "FalconProcData"() -> (w1364:u8[])
                    n4894 = local write "SaveFalconProc"(FALSE ("SaveFalconProc")) -> ()
                    n4895 = Build Path(base path=w1367, name or relative path="FalconProcessed") -> (appended path=w1365:path)
                    n4896 = call "WriteFalconProcessed.vi"("Path:~\\syslogs\\FalconProcessed"=w1365, "FalconProcessedData"=w1364) -> ()  [unwired: 13 in, 1 out]
                    "LastProcSavedID" <- w1363
                    "FalconProcTimeStamp" <- w1362
                  }
                }
              }
            }
            n4897 = Wait Until Next ms Multiple(millisecond multiple=u32 1000) -> ()  [unwired: 1 out]
            n4898 = local read "Quit"() -> (w1226:bool)
          }
          "Archivage SAOMM" <- w950
          n4899 = while {
            stop <- w961 stop-if-true
            n4900 = local read "Cx"() -> (w963:bool)
            n4901 = case shown="False" w963 {
              selector: w963 -> [_ w989]
              tunnel: [w979 w989] -> w962
              frame False {
                # "Si on n'est pas connecté, on fait une tentative ..."
                n4902 = flat-sequence {
                  tunnel: [w980] -> w978
                  tunnel: [w982] -> w979
                  tunnel: w978 -> [_]
                  frame #0 {
                    n4903 = local read "cRIO_commID"() -> (w981:refnum<k5>)
                    n4904 = TCP Close Connection(connection ID=w981) -> (error out=w980:errorcluster)  [unwired: 2 in, 1 out]
                  }
                  frame #1 {
                    n4905 = local read "cRIO address"() -> (w984:string)
                    n4906 = TCP Open Connection(address=w984, remote port or service name=u16 8088, timeout ms (60000)=5000) -> (connection ID=w983:refnum<k5>, error out=w987:errorcluster)  [unwired: 2 in]
                    n4907 = local write "cRIO_commID"(w983) -> ()
                    n4908 = Unbundle By Name(w987) -> ("status"=w986:bool)
                    n4909 = Not(x=w986) -> (.not. x?=w982:bool)
                    n4910 = local write "Cx"(w982) -> ()
                  }
                }
              }
              frame True {
              }
            }
            n4911 = case shown="True" w962 {
              frame False {
                w964 = 0.0 ("indic-T-out")
                n4912 = local write "indic-Tm"(w964) -> ()
                n4913 = local write "indic-T-struct"(w964) -> ()
                n4914 = local write "indic-T-out"(w964) -> ()
                n4915 = local write "indic-T-in"(w964) -> ()
                n4916 = local write "indic-H-out"(w964) -> ()
                n4917 = local write "indic-H-in"(w964) -> ()
              }
              frame True {
                n4918 = local read "cRIO_commID"() -> (w976:refnum<k5>)
                n4919 = call "TCP-read.vi"("timeout (5000)"=60000, "connection ID"=w976) -> ("error out"=w968:errorcluster, "data out"=w977:string)  [unwired: 1 in, 1 out]
                n4920 = Unbundle By Name(w968) -> ("status"=w967:bool)
                n4921 = call "line2array.vi"("data-line"=w977) -> ("data-array"=w975:dbl[])  [unwired: 2 out]
                n4922 = Not(x=w967) -> (.not. x?=w966:bool)
                n4923 = local write "Cx"(w966) -> ()
                n4924 = Index Array(array=w975) -> (element #1=→"indic-T-out":dbl, element #2=→"indic-H-out":dbl, element #3=→"indic-T-in":dbl, element #4=→"indic-H-in":dbl, element #7=→"indic-Tm":dbl, element #8=→"indic-T-struct":dbl)  [unwired: 9 in, 3 out]
              }
            }
            n4925 = local read "Quit"() -> (w961:bool)
          }
          n4926 = while {
            tunnel: [w1147] -> w951
            stop <- w1147 stop-if-true
            # "ErrorDEC en Secondes d'arc ...."
            # "ErrorRA en Secondes d'arc ...."
            # "Applique la correction si le délai est respecté et\nque la valeur de l'erreur totale est plus grande que\nle treshold."
            # "Évalue s'il faut envoyer une commande au relais de guidage.\nEn fonction du mode choisi ..."
            n4927 = local read "Mode"() -> (w1158:u16)
            n4928 = local read "Servo"() -> (w1157:bool)
            n4929 = case shown="0, 1" w1158 {
              tunnel: [w1160 w1163 w1179] -> w1154
              tunnel: [w1160 w1162 w1180] -> w1155
              tunnel: [FALSE w1175 w1187] -> w1146
              frame Default {
                w1160 = 0.0 ("mean")
              }
              frame 0, 1 {
                # "Oh, c'est pas propre ici ... le (-1) a été mis parce\nque comme un gros épais ... j'ai inversé RA/DEC et\nNS/EW dans l'autre boucle ..."
                # "Ne marchera pour une étoile qui serait près de RA=00h00m00s ou RA=23h59m59s"
                # "Opération Fixe ou Asservissement Passif"
                n4930 = local read "GuiderAstrom"() -> (w1172:T4)
                n4931 = local read "LastProcID"() -> (w1176:u64)
                n4932 = local read "CorrID"() -> (w1177:u64)
                n4933 = local read "XCentroid"() -> (w1174:dbl)
                n4934 = local read "YCentroid"() -> (w1173:dbl)
                n4935 = local read "XReference"() -> (w1171:dbl)
                n4936 = local read "YReference"() -> (w1170:dbl)
                n4937 = Greater?(x=w1176, y=w1177) -> (0:w1175:bool)
                n4938 = expression code="x/180.0"(3.141592653589793) -> (w1164:dbl)
                n4939 = call "xy2ad.vi"("Y (px)"=w1170, "X (px)"=w1171, "Astrometry"=w1172) -> ("DEC (°)"=w1167:dbl, "RA (°)"=w1168:dbl)  [unwired: 5 in, 2 out]
                n4940 = call "xy2ad.vi"("Y (px)"=w1173, "X (px)"=w1174, "Astrometry"=w1172) -> ("DEC (°)"=w1165:dbl, "RA (°)"=w1166:dbl)  [unwired: 5 in, 2 out]
                n4941 = case shown="True" w1175 {
                  tunnel: w1176 -> [_ w1178]
                  frame False {
                  }
                  frame True {
                    "CorrID" <- w1178
                  }
                }
                n4942 = formula code="ErrorRA=(CenRA-RefRA)*3600.0*cos(RefDEC*PIsur180);\nErrorDEC=(CenDEC-RefDEC)*3600.0;"("RefRA"=w1168, "RefDEC"=w1167, "CenRA"=w1166, "CenDEC"=w1165, "PIsur180"=w1164) -> ("ErrorRA"=w1163:dbl, "ErrorDEC"=w1162:dbl)
              }
              frame 2 {
                # "Ajouter une condition sur la dérivée locale ???"
                # "Asservissement Actif (LUT + Servo + Guidage)"
                # "Pas besoin d'appliquer la rotation puisque\nseul l'écart de l'hexapode est considéré."
                n4943 = local read "EcartX"() -> (w1181:dbl)
                n4944 = local read "EcartY"() -> (w1184:dbl)
                n4945 = Absolute Value(x=w1181) -> (abs(x)=w1186:dbl)
                n4946 = Absolute Value(x=w1184) -> (abs(x)=w1185:dbl)
                n4947 = Greater Or Equal?(x=w1186, y="CorrTreshold") -> (x >= y?=w1188:bool)
                n4948 = Less?(x="CorrTreshold", y=w1185) -> (x < y?=w1189:bool)
                n4949 = Or(x=w1188, y=w1189) -> (x .or. y?=w1187:bool)
                n4950 = Multiply(x=w1181, y="HexXRate") -> (x*y=w1180:dbl)
                n4951 = Multiply(x="HexYRate", y=w1184) -> (x*y=w1179:dbl)
              }
            }
            n4952 = Tick Count (ms)() -> (millisecond timer value=w1149:u32)
            n4953 = Subtract(x=w1149, y="LastCorr") -> (x-y=w1151:u32)
            n4954 = Greater?(x=w1151, y="CorrDelay") -> (0:w1153:bool)
            n4955 = local read "SNRtreshold"() -> (w1144:dbl)
            n4956 = local read "SNR"() -> (w1145:dbl)
            n4957 = Greater Or Equal?(x=w1145, y=w1144) -> (x >= y?=w1143:bool)
            n4958 = Compound Arithmetic op=AND(w1146, w1143, w1153, w1157) -> (w1148:bool)
            n4959 = case shown="True" w1148 {
              tunnel: w1155 -> [_ w1222]
              tunnel: w1154 -> [_ w1221]
              tunnel: "Corr%" -> [_ w1223]
              frame False {
              }
              frame True {
                # "millisecond d'activation\ndes relais ..."
                # "À déterminer sur l'ordinateur de BonOMM à OMM"
                n4960 = Tick Count (ms)() -> (millisecond timer value=w1225:u32)
                n4961 = formula code="EW=(agg/100)*corrX*rRA;\nNS=(agg/100)*corrY*rDEC;"("agg"=w1223, "rRA"="RateRA", "bRA"="BacklashRA", "rDEC"="RateDEC", "bDEC"="BacklashDEC", "corrX"=w1221, "corrY"=w1222) -> ("NS"=w1220:dbl, "EW"=w1219:dbl)
                n4962 = local write "LastCorr"(w1225) -> ()
                n4963 = local read "path_trackfile"() -> (w1206:path)
                n4964 = control-ref of="GuidingCancel"() -> (w1210:refnum<vi>)
                n4965 = control-ref of="GuideNorth"() -> (w1211:refnum<vi>)
                n4966 = control-ref of="GuideSouth"() -> (w1212:refnum<vi>)
                n4967 = control-ref of="GuideEast"() -> (w1209:refnum<vi>)
                n4968 = control-ref of="GuideWest"() -> (w1208:refnum<vi>)
                n4969 = Strip Path(path=w1206) -> (stripped path=w1204:path)  [unwired: 1 out]
                n4970 = Round To Nearest(number=w1219) -> (nearest integer value=w1216:dbl)
                n4971 = Bundle("GuidingCancel"=w1210, "GuideNorth"=w1211, "GuideSouth"=w1212, "GuideEast"=w1209, "GuideWest"=w1208) -> (w1207:T60)  [unwired: 1 in]
                n4972 = Round To Nearest(number=w1220) -> (nearest integer value=w1217:dbl)
                n4973 = Build Path(base path=w1204, name or relative path="Relays") -> (appended path=w1191:path)
                n4974 = local read "RotationTCS"() -> (w1199:dbl)
                n4975 = local read "ErrX"() -> (w1197:string)
                n4976 = local read "ErrY"() -> (w1196:string)
                n4977 = local read "exptime"() -> (w1198:dbl)
                n4978 = To Long Integer(number=w1217) -> (32bit integer=w1200:i32)
                n4979 = To Long Integer(number=w1216) -> (32bit integer=w1201:i32)
                n4980 = Fract/Exp String To Number(string=w1197) -> (number=w1195:dbl)  [unwired: 3 in, 1 out]
                n4981 = Fract/Exp String To Number(string=w1196) -> (number=w1194:dbl)  [unwired: 3 in, 1 out]
                n4982 = local read "HexX"() -> (w1193:dbl)
                n4983 = local read "HexY"() -> (w1192:dbl)
                n4984 = call "LogRelayData.vi"("Path"=w1191, "XCorr"=w1200, "YCorr"=w1201, "Rotation"=w1199, "Texp"=w1198, "CenX"=w1195, "CenY"=w1194, "XHex"=w1193, "YHex"=w1192) -> ()  [unwired: 7 in]
                n4985 = call "DIO-ApplyCorrection.vi"("TaskCluster"=T21 {"North Task"="Nord", "West Task"="Sud", "South Task"="Est", "East Task"="Ouest"}, "NordSud(ms)"=w1200, "EstOuest(ms)"=w1201, "ReferenceCluster"=w1207) -> ("GuiderRA Error"=w1203:errorcluster, "GuiderDEC Error"=w1202:errorcluster)  [unwired: 10 in]
                n4986 = call "LogRelayError.vi"("Path"=w1191, "GuiderRA Error"=w1203, "GuiderDEC Error"=w1202) -> ()  [unwired: 13 in]
              }
            }
            n4987 = local read "Quit"() -> (w1147:bool)
            n4988 = Wait Until Next ms Multiple(millisecond multiple=u32 50) -> ()  [unwired: 1 out]
          }
          "Guidage" <- w951
          n4989 = while {
            tunnel: [w2561] -> w945
            stop <- w2561 stop-if-true
            # "Boucle de gestions des clients et des commandes SÉRIE et TCP/IP"
            n4990 = stacked-sequence {
              frame #0 {
                # "Vérifie les demandes de connexions en déconnectant :\n  - celles qui sont inactives depuis plus d'une heure\n  x celles dont le client est le même (ne retient que la plus récente)\n  x celles ne provenant pas de 132.204.xxx.xxx"
                n4991 = String To IP(1:"Address du serveur") -> (0:w2568:u32)
                n4992 = call <vilib>:"TCP Listen.vi"("resolve remote address (T)"=FALSE, "net address"=w2568, "timeout ms (wait forever: -1)"=10, "port"="Port Local") -> ("error out"=w2563:errorcluster, "remote port"=w2566:u16, "remote address"=w2564:string, "connection ID"=w2565:refnum<k5>)  [unwired: 3 in, 1 out]
                n4993 = Not Equal?(x=w2564, y="") -> (x != y?=w2567:bool)
                n4994 = case shown="True" w2567 {
                  tunnel: w2566 -> [_ w2575]
                  tunnel: w2565 -> [_ w2578]
                  tunnel: w2564 -> [_ w2574]
                  frame False {
                  }
                  frame True {
                    # "Ne conserve que l'adresse"
                    n4995 = local read "Clients"() -> (w2577:string[])
                    n4996 = for {
                      tunnel: w2577 -> [w2582] mode=indexing
                      tunnel: [w2581] -> w2576 mode=indexing
                      n4997 = Search/Split String(string=w2582, search string/char (-)=":") -> (substring before match=w2581:string)  [unwired: 1 in, 2 out]
                    }
                    n4998 = Search 1D Array(1D array=w2576, element=w2574) -> (index of element=w2573:i32)  [unwired: 1 in]
                    n4999 = Less Than 0?(x=w2573) -> (x < 0?=w2579:bool)
                    n5000 = case shown="False" w2579 {
                      tunnel: w2577 -> [w2595 w2619]
                      tunnel: w2578 -> [w2597 w2610]
                      tunnel: w2575 -> [w2596 w2622]
                      tunnel: w2574 -> [w2584 w2618]
                      tunnel: w2573 -> [_ w2612]
                      frame True {
                        # "l'adresse n'existe pas encore ..."
                        n5001 = Spreadsheet String To Array(delimiter (Tab)=".", format string="%s", spreadsheet string=w2584, array type (2D Dbl)=string[] []) -> (array=w2593:string[])
                        n5002 = Index Array(array=w2593) -> (element #1=w2591:string, element #2=w2590:string)  [unwired: 2 in]
                        n5003 = Equal?(x="132", y=w2591) -> (x = y?=w2587:bool)
                        n5004 = Equal?(x=w2590, y="204" ("x")) -> (x = y?=w2586:bool)
                        n5005 = And(x=w2587, y=w2586) -> (x .and. y?=w2585:bool)
                        n5006 = case shown="True" w2585 {
                          tunnel: w2597 -> [w2599 w2609]
                          tunnel: w2596 -> [_ w2605]
                          tunnel: w2595 -> [_ w2602]
                          tunnel: w2584 -> [_ w2600]
                          frame False {
                            n5007 = TCP Close Connection(connection ID=w2599) -> (error out=w2598:errorcluster)  [unwired: 2 in, 1 out]
                            n5008 = local write "TCP/IP Error"(w2598) -> ()
                          }
                          frame True {
                            n5009 = local read "Clients ID"() -> (w2608:refnum<k5>[])
                            n5010 = Number To Decimal String(number=w2605) -> (decimal integer string=w2604:string)  [unwired: 1 in]
                            n5011 = Insert Into Array(array=w2608, new element=w2609) -> (→"Clients ID":refnum<k5>[])  [unwired: 1 in]
                            n5012 = Concatenate Strings(w2600, ":" ("string"), w2604) -> (w2603:string)
                            n5013 = Insert Into Array(array=w2602, new element=w2603) -> (→"Clients":string[])  [unwired: 1 in]
                          }
                        }
                      }
                      frame False {
                        n5014 = local read "Clients ID"() -> (w2613:refnum<k5>[])
                        n5015 = Number To Decimal String(number=w2622) -> (decimal integer string=w2621:string)  [unwired: 1 in]
                        n5016 = Index Array(array=w2613, index=w2612) -> (element=w2611:refnum<k5>)
                        n5017 = Concatenate Strings(w2618, ":" ("string"), w2621) -> (w2620:string)
                        n5018 = TCP Close Connection(connection ID=w2611) -> (error out=w2615:errorcluster)  [unwired: 2 in, 1 out]
                        n5019 = Replace Array Subset(array=w2619, new element=w2620, index=w2612) -> (w2614:string[])
                        n5020 = local write "TCP/IP Error"(w2615) -> ()
                        n5021 = local write "Clients"(w2614) -> ()
                        n5022 = Replace Array Subset(array=w2613, new element=w2610, index=w2612) -> (w2616:refnum<k5>[])
                        n5023 = local write "Clients ID"(w2616) -> ()
                      }
                    }
                  }
                }
                n5024 = local write "TCP/IP Error"(w2563) -> ()
              }
              frame #1 {
                # "Prends quelques millisecondes pour ramasser des commandes sur les ports ..."
                n5025 = flat-sequence {
                  frame #0 {
                    n5026 = control-ref of="FIFO actif"() -> (w2623:refnum<vi>)
                    n5027 = call "Fifo-Wait4Flag.vi"("Raise Flag ?"=TRUE, "Ctl Refnum IN"=w2623) -> ()  [unwired: 8 in, 2 out]
                  }
                  frame #1 {
                    # "Délai de réception pour chaque client (ms)"
                    n5028 = local read "Excmd VRN"() -> (w2633:refnum<visa-resource-name>)
                    n5029 = local read "TCP/IP Error"() -> (w2632:errorcluster)
                    n5030 = local read "Excom Error"() -> (w2625:errorcluster)
                    n5031 = local read "Clients ID"() -> (w2630:refnum<k5>[])
                    n5032 = local read "CmdFIFO"() -> (w2629:T14)
                    n5033 = call "WaitForCMD.vi"("Clients ID IN"=w2630, "Cmd FIFO IN"=w2629, "TCP/IP Error IN"=w2632, "Excmd VRN"=w2633, "Serial Error IN"=w2625, "Timeout"=u32 20) -> ("Cmd FIFO OUT"=→"CmdFIFO":T61, "TCP/IP Error"=w2631:errorcluster, "Serial Error"=w2626:errorcluster)  [unwired: 7 in]
                    n5034 = local write "TCP/IP Error"(w2631) -> ()
                    n5035 = local write "Excom Error"(w2626) -> ()
                  }
                  frame #2 {
                    n5036 = local write "FIFO actif"(FALSE) -> ()
                  }
                }
              }
            }
            n5037 = local read "Quit"() -> (w2561:bool)
          }
          "Scripts Listener" <- w945
          n5038 = while {
            tunnel: [w2635] -> w946
            stop <- w2635 stop-if-true
            # "Boucle pour la gestion des pop-up et autres événements non-synchronisés"
            n5039 = Array Size(array="FIFO d'erreur") -> (size(s)=w2639:i32)
            n5040 = Greater Than 0?(x=w2639) -> (x > 0?=w2638:bool)
            n5041 = case shown="True" w2638 {
              tunnel: "FIFO d'erreur" -> [_ w2642]
              frame False {
              }
              frame True {
                n5042 = Delete From Array(array=w2642, length=1, index=0) -> (deleted portion=w2643:T7, array with subset deleted=w2641:T7)
                n5043 = local write "FIFO d'erreur"(w2641) -> ()
                n5044 = Index Array(array=w2643) -> (element=w2640:T62)  [unwired: 1 in]
                n5045 = Unbundle By Name(w2640) -> ("Source"=w2646:string)
                n5046 = case shown="\"Hexapod\"" w2646 {
                  tunnel: w2640 -> [w2647 w2650 w2651 w2653 w2655 _]
                  frame "PrAMS" {
                    n5047 = Unbundle By Name(w2647) -> ("Comment"=w2648:string)
                    n5048 = One Button Dialog(message=w2648) -> ()  [unwired: 1 in, 1 out]
                  }
                  frame "Hexapod" {
                    n5049 = Unbundle By Name(w2650) -> ("Comment"=w2649:string)
                    n5050 = One Button Dialog(message=w2649) -> ()  [unwired: 1 in, 1 out]
                  }
                  frame "offset" {
                    # "Error Code\nb0 : 01 : Erreur mineure\nb1 : 02 : Intervention nécessaire\nb2 : 04 : Erreur avec TCS\nb3 : 08 : Erreur avec Tables\nb4 : 16 : Erreur avec MaximDL\nb5 : 32 : Erreur avec Périphérique\nb6 : 64 : Erreur Majeure\nb7 : 128 : Commande inexistante"
                    # "Warning Code\nb0 : 01 : Micro-Offset non effecuté (pas de guidage)\nb1 : 02 : Guidage non-redémarré, référence perdue\nb2 : 04 : Erreur avec TCS\nb3 : 08 : Erreur avec Tables\nb4 : 16 : Erreur MaximDL/Caméra de guidage\nb5 : 32 : \nb6 : 64 : Erreur avec la base de données USNO\nb7 : 128 : Impossible d'arrêter le télescope ou les tables de guidages !!!"
                    n5051 = call "Offset_Error&Warnings.vi"("Cluster"=w2651) -> ()  [unwired: 6 in]
                  }
                  frame "ETCS" {
                    # "Écrit le commentaire directement dans le dialog"
                    n5052 = Unbundle By Name(w2653) -> ("Comment"=w2652:string)
                    n5053 = One Button Dialog(message=w2652) -> ()  [unwired: 1 in, 1 out]
                  }
                  frame "TCS" {
                    n5054 = Unbundle By Name(w2655) -> ("Comment"=w2654:string)
                    n5055 = One Button Dialog(message=w2654) -> ()  [unwired: 1 in, 1 out]
                  }
                  frame Default {
                    # "Source de l'erreur indéfinie ..."
                  }
                }
              }
            }
            n5056 = Wait (ms)(milliseconds to wait=u32 50) -> ()  [unwired: 1 out]
            n5057 = local read "Quit"() -> (w2635:bool)
          }
          "Afficahge d'erreur" <- w946
          n5058 = while {
            tunnel: [w2768] -> w944
